vi "DB_SelectSumStats.vi"(8 "error in (no error)":errorcluster, 11 "SQLite Connection in":refnum<class "Connection.lvclass">) -> (0 "error out":errorcluster, 1 "Array":i64[](array[numeric]), 3 "SQLite Connection":refnum<class "Connection.lvclass">)   [LabVIEW 2020]
doc: "Returns how many times each option was chosen using SUM SQL statement."
uses:
  <vilib>/drjdpowell/SQLite Library/SQL Connection/Connection.lvclass
  <vilib>/drjdpowell/SQLite Library/SQL Statement/SQL Statement.lvclass/SQL Statement.ctl
  <vilib>/drjdpowell/SQLite Library/SQL Statement/Column I64.vi
  <vilib>/drjdpowell/SQLite Library/SQL Statement/Error Message.vi
  <vilib>/drjdpowell/SQLite Library/SQL Statement/SQL Statement.lvclass
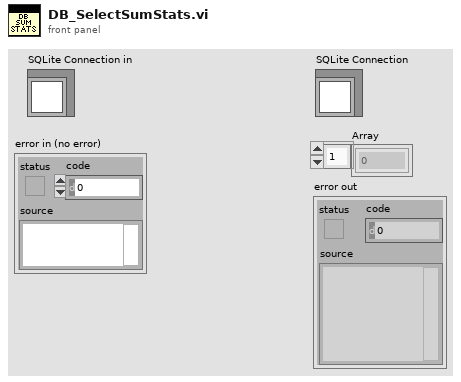
[diagram p1: front panel]
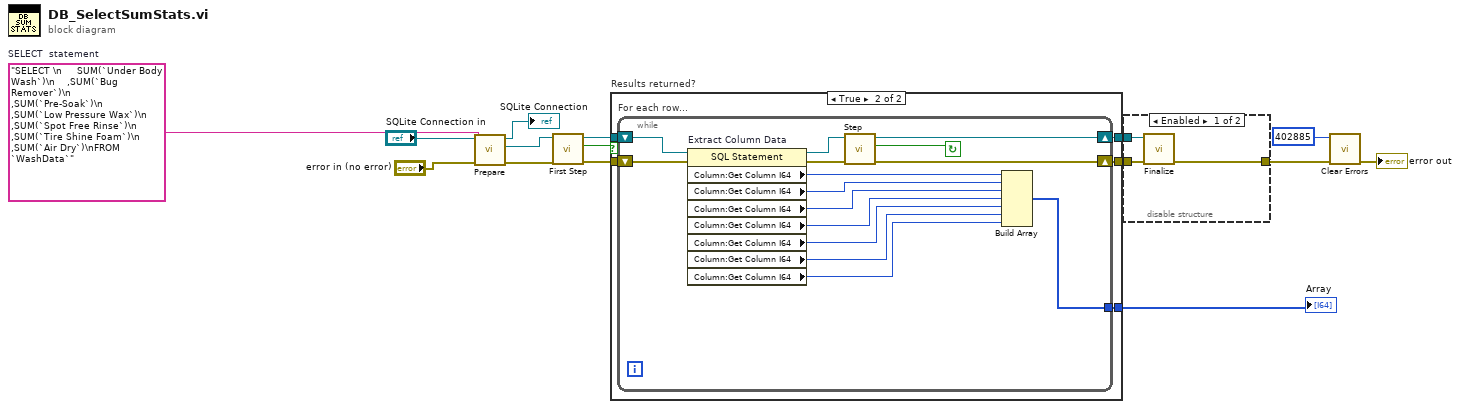
[diagram p0: block diagram]
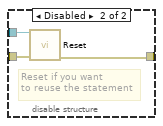
[diagram p2: hidden frame]
diagram:
  w13 = "SELECT \n     SUM(`Under Body Wash`)\n    ,SUM(`Bug Remover`)\n    ,SUM(`Pre-Soak`)\n    ,SUM(`Low Pressure Wax`)\n    ,SUM(`Spot Free Rinse`)\n    ,SUM(`Tire Shine Foam`)\n    ,SUM(`Air Dry`)\nFROM `WashData`"  # SELECT  statement
  n1 = call <vilib>:"Prepare.vi"("error in (no error)"="error in (no error)", "SQL"=w13, "SQLite Connection in"="SQLite Connection in") -> ("error out"=w9:errorcluster, "SQL Statement"=w8:refnum<class "SQL Statement.lvclass">, "SQLite Connection"=→"SQLite Connection":refnum<class "Connection.lvclass">)  [unwired: 4 in, 2 out]
  n2 = call <vilib>:"First Step.vi"("error in (no error)"=w9, "SQL Statement in"=w8) -> ("error out"=w11:errorcluster, "Row returned"=w10:bool, "SQL Statement"=w12:refnum<class "SQL Statement.lvclass">)  [unwired: 7 in]
  n3 = case "Results returned?" shown="True" w10 {
    tunnel: [w17 w22] -> w14
    tunnel: [w16 w21] -> w15
    tunnel: w12 -> [w17 w20]
    tunnel: w11 -> [w16 w19]
    tunnel: [_ w18] -> w4
    frame False {
    }
    frame True {
      n4 = while "For each row..." {
        shift-right: [w36] -> w22
        shift-left: w20 -> [w33]
        shift-right: [w34] -> w21
        shift-left: w19 -> [w32]
        tunnel: [w28] -> w18
        stop <- w31 continue-if-true
        n5 = property on="Extract Column Data" class="SQL Statement"(reference=w33, error in=w32) -> (reference out=w37:refnum<class "SQL Statement.lvclass">, error out=w35:errorcluster, "Column:Get Column I64"=w30:i64, "Column:Get Column I64"=w29:i64, "Column:Get Column I64"=w27:i64, "Column:Get Column I64"=w26:i64, "Column:Get Column I64"=w25:i64, "Column:Get Column I64"=w24:i64, "Column:Get Column I64"=w23:i64)
        n6 = call <vilib>:"Step.vi"("error in (no error)"=w35, "SQL Statement in"=w37) -> ("error out"=w34:errorcluster, "Row returned"=w31:bool, "SQL Statement"=w36:refnum<class "SQL Statement.lvclass">)  [unwired: 7 in]
        n7 = Build Array(w30, w29, w27, w26, w25, w24, w23) -> (w28:i64[])
      }
    }
  }
  "Array" <- w4
  n8 = disable-structure "Diagram Disable Structure" shown="Enabled" {
    disable-tunnel: w14 -> [w40 w43]
    disable-tunnel: w15 -> [w39 w42]
    disable-tunnel: [w38 w41] -> w2
    frame Enabled {
      n9 = call <vilib>:"Finalize.vi"("error in (no error)"=w39, "SQL Statement in"=w40) -> ("error out"=w38:errorcluster)  [unwired: 9 in]
    }
    frame Disabled {
      # "Reset if you want\nto reuse the statement"
      n10 = call <vilib>:"Reset.vi"("error in (no error)"=w42, "SQL Statement in"=w43) -> ("error out"=w41:errorcluster)  [unwired: 8 in, 1 out]
    }
  }
  n11 = call <vilib>:"Clear Errors.vi"("error in (no error)"=w2, "specific error code to clear (0: all)"=402885) -> ("error out"=→"error out":errorcluster)  [unwired: 4 in, 1 out]
